vi "Cal-Apply Microphone Correction.vi"(0 "PTC Mag in":dbl[](array[numeric]), 5 "PTC Phase in":dbl[](array[numeric]), 7 "Frequency in":dbl[](array[numeric]), 9 "Correction curve":path, 11 "error in (no error)":errorcluster) -> (4 "PTC Mag out":dbl[](array[numeric]), 6 "PTC Phase out":dbl[](array[numeric]), 8 "Frequency out":dbl[](array[numeric]), 15 "error out":errorcluster)   [LabVIEW 2020]
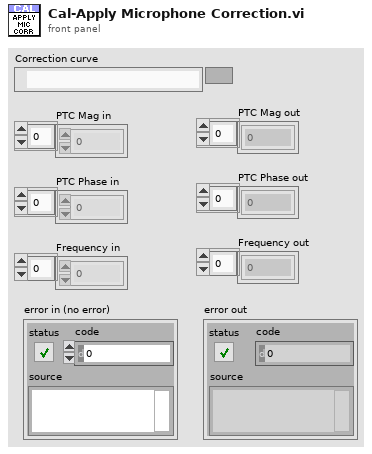
[diagram p1: front panel]
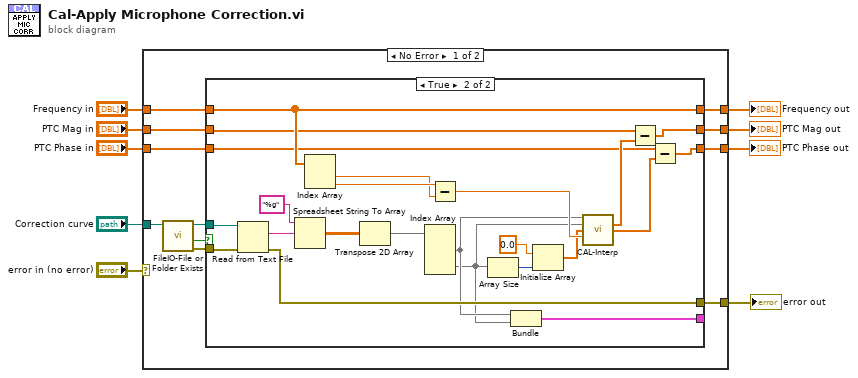
[diagram p0: block diagram]
diagram:
  n1 = case shown="No Error" "error in (no error)" {
    selector: "error in (no error)" -> [_ w48]
    tunnel: "Frequency in" -> [w20 w51]
    tunnel: "Correction curve" -> [w19 _]
    tunnel: [w13 w51] -> w6
    tunnel: [w12 w50] -> w5
    tunnel: "PTC Mag in" -> [w15 w50]
    tunnel: [w11 w49] -> w3
    tunnel: "PTC Phase in" -> [w14 w49]
    tunnel: [w10 w48] -> w1
    frame No Error {
      n2 = call "FileIO-File or Folder Exists.vi"("path"=w19) -> ("error out"=w16:errorcluster, "Exists?"=w17:bool, "dup path"=w18:path)  [unwired: 7 in, 1 out]
      n3 = case shown="True" w17 {
        tunnel: w20 -> [w24 w44]
        tunnel: w18 -> [_ w37]
        tunnel: w16 -> [w21 w36]
        tunnel: w15 -> [w23 w43]
        tunnel: w14 -> [w22 w40]
        tunnel: [w24 w44] -> w13
        tunnel: [w23 w41] -> w12
        tunnel: [w22 w38] -> w11
        tunnel: [w21 w35] -> w10
        tunnel: [_ w26] -> _
        frame False {
        }
        frame True {
          n4 = Read from Text File(file (use dialog)=w37, error in=w36) -> (text=w34:string, error out=w35:errorcluster)  [unwired: 2 in, 2 out]
          n5 = Spreadsheet String To Array(format string="%g", spreadsheet string=w34) -> (array=w33:dbl[][])  [unwired: 2 in]
          n6 = Index Array(array=w44) -> (element #1=w46:dbl, element #2=w47:dbl)  [unwired: 2 in]
          n7 = Transpose 2D Array(2D array=w33) -> (transposed array=w25:dbl[][])
          n8 = Index Array(array=w25) -> (element #1=w28:dbl[], element #2=w27:dbl[])  [unwired: 4 in]
          n9 = Subtract(x=w47, y=w46) -> (x-y=w45:dbl)
          n10 = Array Size(array=w27) -> (size(s)=w32:i32)
          n11 = Bundle(w28, w27) -> (w26:cluster{dbl[], dbl[]})  [unwired: 1 in]
          n12 = Initialize Array(0.0, w32) -> (w30:dbl[])
          n13 = call "CAL-Interp.vi"("Frequency (Hz)"=w28, "Magnitude (dB)"=w27, "Phase (degrees)"=w30, "df (Hz)"=w45) -> ("Interp Magnitude (dB)"=w42:dbl[], "Interp Phase (degrees)"=w39:dbl[])  [unwired: 8 in, 2 out]
          n14 = Subtract(x=w43, y=w42) -> (x-y=w41:dbl[])
          n15 = Subtract(x=w40, y=w39) -> (x-y=w38:dbl[])
        }
      }
    }
    frame Error {
    }
  }
  "Frequency out" <- w6
  "PTC Phase out" <- w3
  "PTC Mag out" <- w5
  "error out" <- w1
